vi "DeleteImaqFromSavedQueue.vi"() -> ()   [LabVIEW 2011]
panel:
  out "saved":i32
  out "dealloc # of images":dbl
  in  "max check time in ms":i32=10000
  out "Bytes in use":u64 format="%.0p"
  in  "Max Bytes Memory":u64=300000000 format="%.0p"
  # "images not saved in temp or in use have access >0"
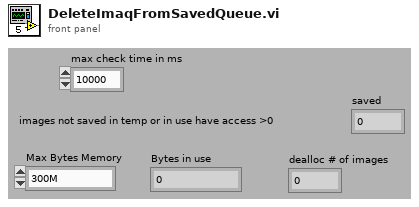
[diagram p1: front panel]
types:
  T1 = enum16{"None/#Datasets", "Clear", "TagValueOf#", "AddValues", "ReadValue", "ChangeValue", "Get all"}
  T2 = enum16{"status", "createIMAQ", "getIMAQ", "getNumber", "deleteIMAQ", "deleteAll", "MemoryUsage", "GetAccess", "DecreaseAccess", "ActualIndex", "ElementToNumber"}
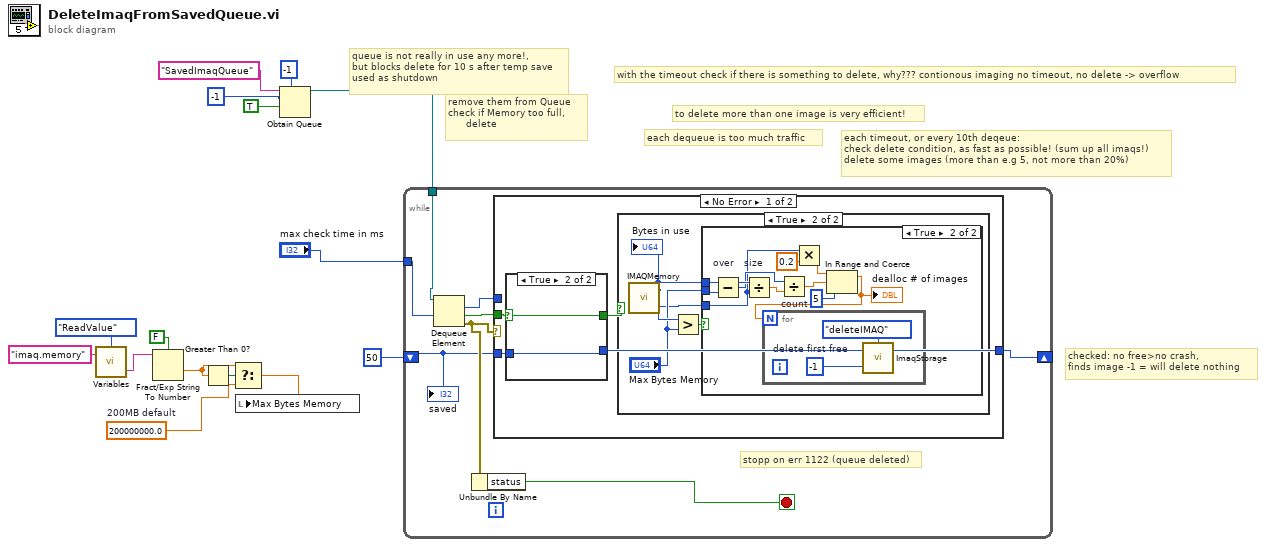
[diagram p0: block diagram]
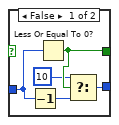
[diagram p2: hidden frame]
diagram:
  w6 = 200000000.0  # 200MB default
  # "each timeout, or every 10th deqeue:\ncheck delete condition, as fast as possible! (sum up all imaqs!)\ndelete some images (more than e.g 5, not more than 20%)"
  # "checked: no free>no crash, \nfinds image -1 = will delete nothing"
  # "each dequeue is too much traffic"
  # "to delete more than one image is very efficient!"
  # "queue is not really in use any more!, \nbut blocks delete for 10 s after temp save\nused as shutdown"
  # "with the timeout check if there is something to delete, why??? contionous imaging no timeout, no delete -> overflow"
  # "remove them from Queue\ncheck if Memory too full, \n      delete"
  n1 = call "Variables.vi"("Tag in"="imaq.memory", "Command"=T1."ReadValue") -> ("value out"=w8:string)  [unwired: 1 in, 2 out]
  n2 = Fract/Exp String To Number(use system decimal point (T)=FALSE ("Systemdezimalzeichen verwenden (T)"), string=w8) -> (number=w3:dbl)  [unwired: 3 out]
  n3 = Greater Than 0?(x=w3) -> (x > 0?=w4:bool)
  n4 = Select(t=w3, s=w4, f=w6) -> (s? t:f=w5:dbl)
  n5 = local write "Max Bytes Memory"(w5) -> ()
  n6 = Obtain Queue(max queue size (-1, unlimited)=-1, name (unnamed)="SavedImaqQueue", element data type=-1, create if not found? (T)=TRUE) -> (queue out=w12:refnum<queue>)  [unwired: 1 in, 2 out]
  n7 = while {
    tunnel: w12 -> [w23]
    tunnel: "max check time in ms" -> [w18]
    shift-right: [w16] -> _
    shift-left: 50 -> [w17]
    stop <- w22 stop-if-true
    # "stopp on err 1122 (queue deleted)"
    n8 = Dequeue Element(queue=w23, timeout in ms (-1)=w18) -> (element=w19:i32, timed out?=w21:bool, error out=w20:errorcluster)  [unwired: 1 in, 1 out]
    n9 = Unbundle By Name(w20) -> ("status"=w22:bool)
    n10 = case shown="No Error" w20 {
      tunnel: w21 -> [w27 _]
      tunnel: w19 -> [_ _]
      tunnel: w17 -> [w25 w51]
      tunnel: [w24 w51] -> w16
      frame No Error {
        n11 = case shown="True" w27 {
          selector: w27 -> [_ w34]
          tunnel: [w32 w34] -> w26
          tunnel: w25 -> [w30 w33]
          tunnel: [w28 w33] -> w24
          frame False {
            n12 = Decrement(x=w30) -> (x-1=w29:i32)
            n13 = Less Or Equal To 0?(x=w30) -> (x <= 0?=w32:bool)
            n14 = Select(t=10, s=w32, f=w29) -> (s? t:f=w28:i32)
          }
          frame True {
          }
        }
        n15 = case shown="True" w26 {
          frame False {
            # "do no check after every saved element"
          }
          frame True {
            n16 = call "IMAQMemory.vi"() -> ("Bytes in use"=w37:u64, "Images in use"=w35:i32)  [unwired: 1 out]
            "Bytes in use" <- w37
            n17 = Greater?(x=w37, y="Max Bytes Memory") -> (0:w38:bool)
            n18 = case shown="True" w38 {
              tunnel: w37 -> [_ w48]
              tunnel: "Max Bytes Memory" -> [_ w47]
              tunnel: w35 -> [_ w42]
              frame False {
                # "enaugh space left"
              }
              frame True {
                n19 = Subtract "over"(x=w48, y=w47) -> (x-y=w46:u64)
                n20 = Divide "size"(x=w48, y=w42) -> (x/y=w45:dbl)
                n21 = Divide "count"(x=w46, y=w45) -> (x/y=w44:dbl)
                n22 = Multiply(x=w42, y=0.2) -> (x*y=w40:dbl)
                n23 = In Range and Coerce(upper limit=w40, x=w44, lower limit=5 ("unterer Grenzwert")) -> (coerced(x)=w39:dbl)  [unwired: 1 out]
                "dealloc # of images" <- w39
                n24 = for {
                  N: w39 -> [_]
                  w50 = -1  # delete first free
                  n25 = call "ImaqStorage.vi"("Number"=w50, "Command"=T2."deleteIMAQ") -> ()  [unwired: 1 in, 2 out]
                }
              }
            }
          }
        }
      }
      frame Error {
        # "end"
      }
    }
    "saved" <- w17
  }
